vi "tx QAM.vi"() -> ()   [LabVIEW 2014]
uses:
  <instrlib>/niUSRP/niUSRP Write Tx Data (CDB Cluster).vi
  <vilib>/addons/Modulation/niDMT.lvlib
panel:
  in  "pulse shaping filter (none)":T1(ring)=enum."Raised Cosine"
  out "output bit stream":i8[](array[numeric])=[1, 1, 1, 1, 1, 1, 1, 0, 1, 0, 0, 0, 1, 0, 1, 1, 0, 0, 0, 1, 1, 1, 0, 1, 0, 1, 1, 0, 0, 1, 0, 1, 1, 0, 0, 1, 1, 1, 1, 0, 0, 0, 1, 1, 1, 1, 1, 0, 1, 1, 1, 0, 1, 0, 0, 0, 0, 0, 1, 1, 0, 1, 0, 1, 1, 0, 1, 1, 0, 1, 1, 1, 0, 1, 1, 0, 0, 0, 0, 0, 1, 0, 1, 1, 0, 1, 0, 1, 1, 1, 1, 1, 0, 1, 0, 1, 0, 1, 0, 1, 0, 0, 0, 0, 0, 0, 1, 0, 1, 0, 0, 1, 0, 1, 0, 1, 1, 1, 1, 0, 0, 1, 0, 1, 1, 1, 0, 1, 1, 1, 0, 0, 0, 0, 0, 0, 1, 1, 1, 0, 0, 1, 1, 1, 0, 1, 0, 0, 1, 0, 0, 1, 1, 1, 1, 0, 1, 0, 1, 1, 1, 0, 1, 0, 1, 0, 0, 0, 1, 0, 0, 1, 0, 0, 0, 0, 1, 1, 0, 0, 1, 1, 1, 0, 0, 0, 0, 1, 0, 1, 1, 1, 1, 0, 1, 1, 0, 1, 1, 0, 0, 1, 1, 0, 1, 0, 0, 0, 0, 1, 1, 1, 0, 1, 1, 1, 1, 0, 0, 0, 0, 1, 1, 1, 1, 1, 1, 1, 1, 1, 0, 0, 0, 0, 0, 1, 1, 1, 1, 0, 1, 1, 1, 1, 1, 0, 0, 0, 1, 0, 1, 1, 1, 0, 0, 1]
  out "Constellation Graph":T2(graph)
  out "error out":errorcluster
  in  "Stop":bool
  in  "active antenna":string="TX1"
  in  "gain":dbl=20.0 format="%#_6f"
  in  "carrier frequency":dbl=434000000.0 format="%#_6p"
  in  "IQ rate":dbl=400000.0 format="%#_6p"
  in  "device names":refnum<k15>="10.100.1.125"
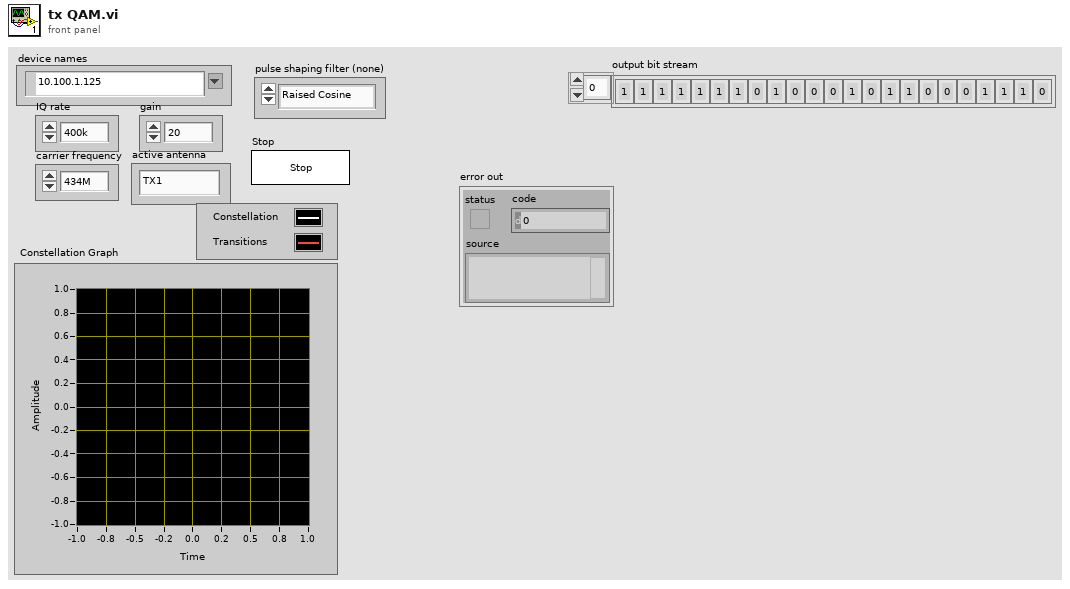
[diagram p1: front panel]
types:
  T1 = enum16{"none", "Raised Cosine", "Root Raised Cos", "Gaussian"}
  T2 = cluster{"constellation":dbl[], "oversampled data":dbl[]}[]
  T3 = typedef "niAMT.lvlib/Complex Data Waveform.ctl" = cluster{"t0":dbl, "dt":dbl, "Y":cdb[]}
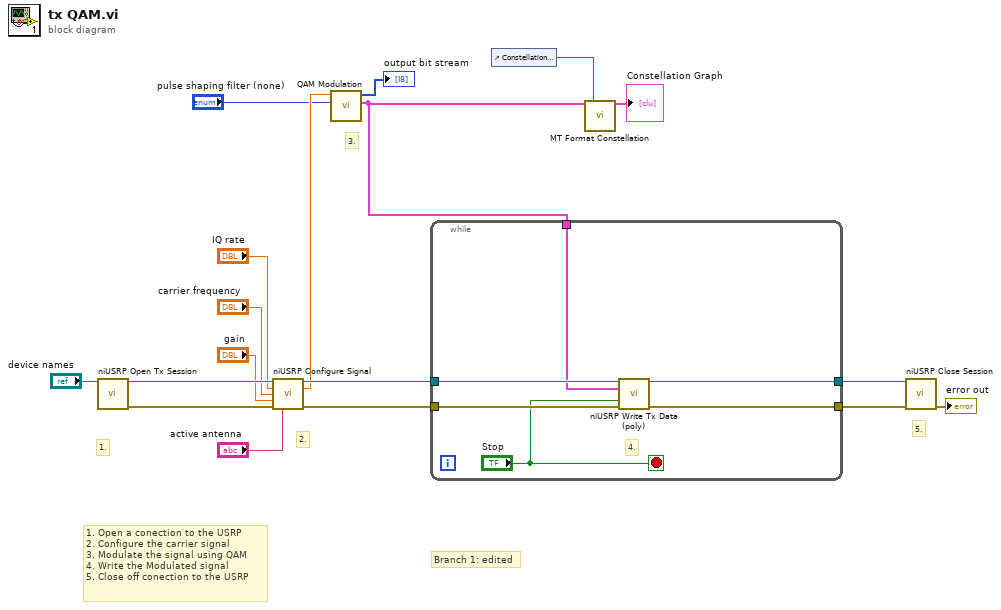
[diagram p0: block diagram]
diagram:
  # "Branch 1: edited"
  # "5."
  # "3."
  # "1. Open a conection to the USRP\n2. Configure the carrier signal\n3. Modulate the signal using QAM\n4. Write the Modulated signal\n5. Close off conection to the USRP"
  # "2."
  # "1."
  n1 = call <instrlib>:"niUSRP Open Tx Session.vi"("device names"="device names") -> ("session handle out"=w18:refnum<k15>, "error out"=w14:errorcluster)  [unwired: 13 in]
  n2 = call <instrlib>:"niUSRP Configure Signal.vi"("session handle"=w18, "IQ rate"="IQ rate", "carrier frequency"="carrier frequency", "gain"="gain", "error in (no error)"=w14, "active antenna"="active antenna") -> ("session handle out"=w8:refnum<k15>, "coerced IQ rate"=w6:dbl, "error out"=w15:errorcluster)  [unwired: 5 in, 2 out]
  n3 = call "QAM Modulation.vi"("pulse shaping filter (none)"="pulse shaping filter (none)", "coerced IQ rate"=w6) -> ("output complex waveform"=w1:T3, "output bit stream"=→"output bit stream":i8[])  [unwired: 8 in]
  n4 = while {
    tunnel: w8 -> [w24]
    tunnel: [w23] -> w17
    tunnel: [w22] -> w16
    tunnel: w15 -> [w21]
    tunnel: w1 -> [w19]
    stop <- "Stop" stop-if-true
    # "4."
    n5 = call-poly <instrlib>:"niUSRP Write Tx Data (poly).vi"("session handle"=w24, "data"=w19, "end of data?"="Stop", "error in (no error)"=w21) -> ("session handle out"=w23:refnum<k15>, "error out"=w22:errorcluster)  [unwired: 10 in]
  }
  n6 = control-ref of="Constellation Graph"() -> (w5:refnum<vi>)
  n7 = call <vilib>:"MT Format Constellation.vi"("waveform"=w1, "constellation reference"=w5) -> ("constellation graph"=→"Constellation Graph":T2)  [unwired: 3 in, 10 out]
  n8 = call <instrlib>:"niUSRP Close Session.vi"("session handle"=w17, "error in (no error)"=w16) -> ("error out"=→"error out":errorcluster)  [unwired: 13 in]
